vi "Indexer.vi"(11 "Output Cluster in":T1) -> ()   [LabVIEW 2015]
uses:
  Joytsick/Controls to Cmmnds Output Clust.ctl
  Joytsick/Controls to Cmmnds Type.ctl
  <vilib>/Rock Robotics/WPI/Relay/WPI_RelayValue.ctl
  Global Vars.vi
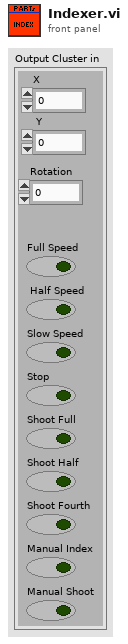
[diagram p1: front panel]
types:
  T1 = typedef "Controls to Cmmnds Output Clust.ctl" = cluster{"X ":dbl, " Y":dbl, "Rotation":dbl, "Full Speed":bool, " Half Speed":bool, "Slow Speed":bool, "Stop":bool, "Shoot Full":bool, "Shoot Half":bool, "Shoot Fourth":bool, "Manual Index":bool, "Manual Shoot":T2}
  T2 = typedef "Controls to Cmmnds Type.ctl" = bool
  T3 = typedef "WPI_RelayValue.ctl" = enum16{"Off", "On", "Forward", "Reverse"}
  T4 = typedef "WPI_RelayDevRef.ctl" = cluster{"DevStatus":errorcluster, "Relay Channel":T5, "Relay Direction":T6}
  T5 = typedef "FPGA_DIORelayChannel.ctl" = enum8{"Relay 0", "Relay 1", "Relay 2", "Relay 3", "Invalid"}
  T6 = typedef "WPI_RelayDirection.ctl" = enum16{"Both directions", "Forward only", "Reverse only"}
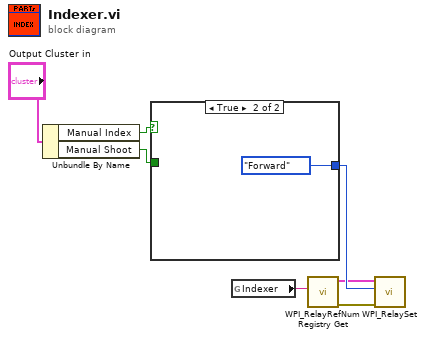
[diagram p0: block diagram]
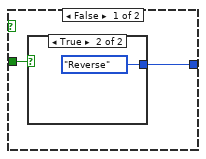
[diagram p2: hidden frame]
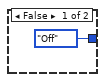
[diagram p3: hidden frame]
diagram:
  n1 = Unbundle By Name("Output Cluster in") -> ("Manual Index"=w5:bool, "Manual Shoot"=w7:T2)
  n2 = case shown="True" w5 {
    tunnel: [w8 WPI_RelayValue."Forward" ("RelayValue")] -> w6
    tunnel: w7 -> [w9 _]
    frame False {
      n3 = case shown="True" w9 {
        tunnel: [WPI_RelayValue."Off" ("RelayValue") WPI_RelayValue."Reverse" ("RelayValue")] -> w8
        frame False {
        }
        frame True {
        }
      }
    }
    frame True {
    }
  }
  n4 = global read "Global Vars.vi" "Indexer"() -> (w2:string)
  n5 = call <vilib>:"WPI_RelayRefNum Registry Get.vi"("refnum name"=w2) -> ("error out"=w4:errorcluster, "RelayDevRef"=w3:T4)  [unwired: 9 in]
  n6 = call <vilib>:"WPI_RelaySet.vi"("error in (no error)"=w4, "RelayValue"=w6, "RelayDevRef"=w3) -> ()  [unwired: 7 in, 2 out]
